vi "H5Literate_by_name.vi"(0 "Location Ref":T1, 1 "Index Type":T3 items=["H5_INDEX_UNKNOWN"=-1, "H5_INDEX_NAME"=0, "H5_INDEX_CRT_ORDER"=1], 2 "Order":T2 items=["H5_ITER_UNKNOWN"=-1, "H5_ITER_INC"=0, "H5_ITER_DEC"=1], 5 "Name":string=".", 7 "User data":variant, 9 "Index":u64, 11 "error in (no error)":errorcluster, 12 "Callback VI Ref":refnum<vi>, 13 "lapl_id":T1) -> (4 "Location Ref out":T1, 8 "User data out":variant, 10 "Index out":u64, 15 "error out":errorcluster)   [LabVIEW 2017]
doc: "Iterates through links in a group."
uses:
  <vilib>/UPVI/lvhdf5/library.llb/HDF5 Ref.ctl
  <vilib>/UPVI/lvhdf5/link.llb/H5L_info_t.ctl
  <vilib>/UPVI/lvhdf5/link.llb/H5L_type_t.ctl
  <vilib>/UPVI/lvhdf5/datatype.llb/H5T_cset_t.ctl
  <vilib>/UPVI/lvhdf5/library.llb/H5_index_t.ctl
  <vilib>/UPVI/lvhdf5/library.llb/H5_iter_order_t.ctl
  <vilib>/UPVI/lvhdf5/h5helper.dll
panel:
  in  "Event Data Type":T7 {"info"."cset" items=["H5T_CSET_ERROR"=-1, "H5T_CSET_ASCII"=0, "H5T_CSET_UTF8"=1]; "info"."type" items=["H5L_TYPE_ERROR"=-1, "H5L_TYPE_HARD"=0, "H5L_TYPE_SOFT"=1, "H5L_TYPE_EXTERNAL"=64, "H5L_TYPE_MAX"=255]}
  # "LVHDF5 Toolkit\nCopyright (c) 2005-2013 by Jason D. Sommerville\nCopyright (c) 2014-2015 by UPVI, LLC.\n\nThis use and distribution of this file is governed by the terms found in \nLICENSE.txt distributed with this toolkit and installed at\n <user.lib>\\_lvhdf5\\LICENSE.txt"
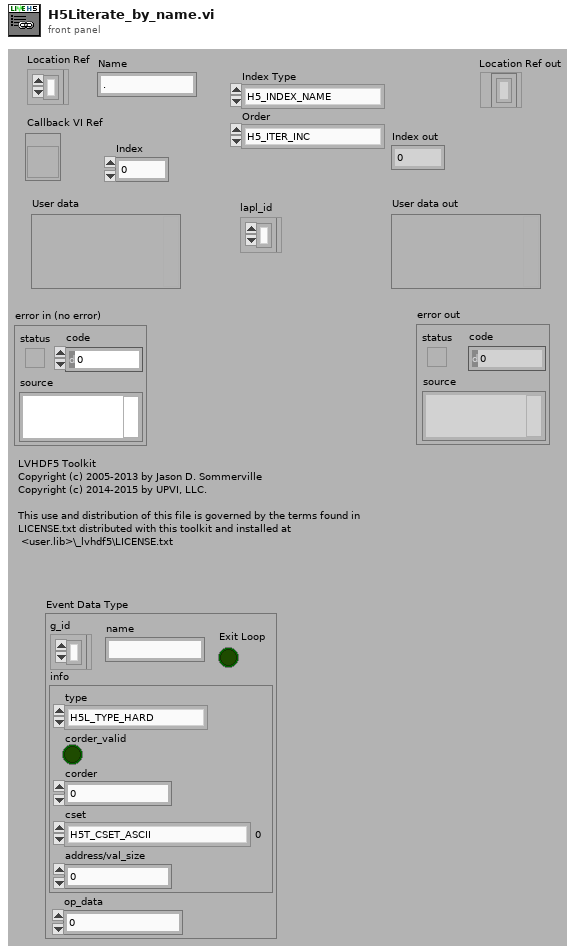
[diagram p1: front panel]
types:
  T1 = typedef "HDF5 Ref.ctl" = refnum<k1>
  T2 = typedef "H5_iter_order_t.ctl" = i32
  T3 = typedef "H5_index_t.ctl" = i32
  T4 = typedef "H5L_info_t.ctl" = cluster{"type":T5, "corder_valid":bool, "corder":i64, "cset":T6, "address/val_size":u64}
  T5 = typedef "H5L_type_t.ctl" = i32
  T6 = typedef "H5T_cset_t.ctl" = i32
  T7 = cluster{"g_id":T1, "name":string, "info":T4, "Exit Loop":bool, "op_data":u64}
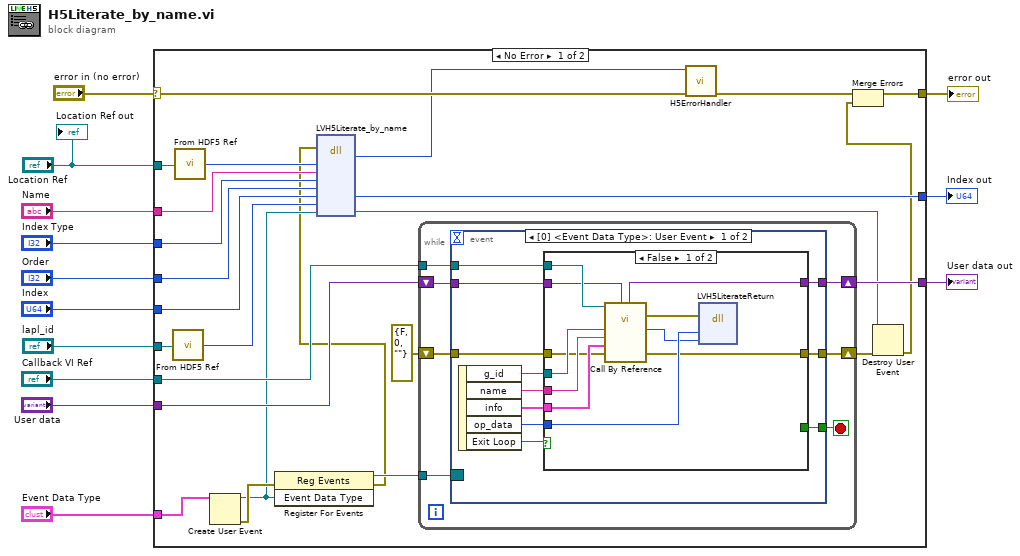
[diagram p0: block diagram]
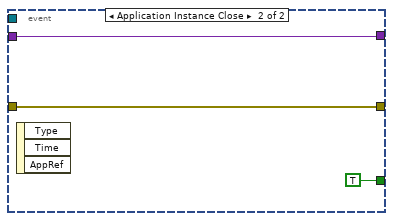
[diagram p3: hidden frame]
diagram:
  n1 = case shown="No Error" "error in (no error)" {
    selector: "error in (no error)" -> [w38 w76]
    tunnel: [w24 w76] -> w12
    tunnel: "Location Ref" -> [w36 _]
    tunnel: "Callback VI Ref" -> [w34 _]
    tunnel: "User data" -> [w33 w75]
    tunnel: "Event Data Type" -> [w30 _]
    tunnel: [w31 w75] -> w8
    tunnel: "Index" -> [w27 w74]
    tunnel: [w26 w74] -> w5
    tunnel: "Index Type" -> [w20 _]
    tunnel: "Order" -> [w19 _]
    tunnel: "Name" -> [w18 _]
    tunnel: "lapl_id" -> [w17 _]
    frame No Error {
      n2 = call <vilib>:"From HDF5 Ref.vi"("HDF5 Ref"=w17) -> ("I32"=w16:i32)
      n3 = call <vilib>:"From HDF5 Ref.vi"("HDF5 Ref"=w36) -> ("I32"=w28:i32)
      n4 = Create User Event(user event datatype=w30) -> (user event=w29:refnum<user-event>, error out=w35:errorcluster)  [unwired: 1 in]
      n5 = register-events(error in=w35, w29) -> (reference out=w32:refnum<event-registration>, error out=w15:errorcluster)  [unwired: 1 in]
      n6 = dll-call lib="C:/Program Files/National Instruments/LabVIEW 2017/vi.lib/UPVI/lvhdf5/h5helper.dll" fn="LVH5Literate_by_name"(error in=w15, "grp_id"=w28, "grp_name"=w18, "index_type"=w20, "order"=w19, "idx"=w27, "lapl_id"=w16, "lvevt"=w29) -> ("return type"=w37:i32, "idx"=w26:u64, "lvevt"=w21:refnum<user-event>)  [unwired: 7 in, 2 out]
      n7 = while {
        tunnel: w32 -> [w45]
        tunnel: w34 -> [w44]
        shift-right: [w42] -> w31
        shift-left: w33 -> [w43]
        shift-right: [w40] -> w23
        shift-left: errorcluster {"status"=FALSE, "code"=0, "source"=""} ("error out") -> [w39]
        stop <- w41 stop-if-true
        n8 = event shown="[0] <Event Data Type>: User Event" {
          selector: w45 -> [_ _]
          dyn-events: _ -> [_ _]
          timeout: _ -> [_ _]
          tunnel: w44 -> [w56 _]
          tunnel: w43 -> [w52 w72]
          tunnel: [w51 w72] -> w42
          tunnel: [w50 TRUE] -> w41
          tunnel: [w47 w71] -> w40
          tunnel: w39 -> [w46 w71]
          event User Event {
            n9 = event-data() -> ("g_id"=w55:T1, "name"=w54:string, "info"=w53:T4, "op_data"=w48:u64, "Exit Loop"=w49:bool)  [unwired: 1 in]
            n10 = case shown="False" w49 {
              selector: w49 -> [_ w69]
              tunnel: w56 -> [w67 _]
              tunnel: w55 -> [w66 _]
              tunnel: w54 -> [w65 _]
              tunnel: w53 -> [w64 _]
              tunnel: w52 -> [w63 w70]
              tunnel: [w62 w70] -> w51
              tunnel: [_ w69] -> w50
              tunnel: w48 -> [w60 _]
              tunnel: [w58 w68] -> w47
              tunnel: w46 -> [w57 w68]
              frame False {
                n11 = call-by-ref "?"(reference=w67, "op_data"=w63, "error in (no error)"=w57, "info"=w64, "name"=w65, "g_id"=w66) -> (error out=w61:errorcluster, 0:"error out"=w58:errorcluster, "Stop"=w59:i32, "op_data out"=w62:variant)  [unwired: 5 in, 1 out]
                n12 = dll-call lib="C:/Program Files/National Instruments/LabVIEW 2017/vi.lib/UPVI/lvhdf5/h5helper.dll" fn="LVH5LiterateReturn"(error in=w61, "op_data"=w60, "result"=w59) -> ()  [unwired: 5 in, 2 out]
              }
              frame True {
              }
            }
          }
          event Application Instance Close {
            n13 = event-data() -> ()  [unwired: 1 in, 3 out]
          }
        }
      }
      n14 = call <vilib>:"H5ErrorHandler.vi"("error in (no error)"=w38, "herr_t"=w37) -> ("error out"=w25:errorcluster)  [unwired: 3 in, 4 out]
      n15 = Destroy User Event(user event=w21, error in=w23) -> (error out=w22:errorcluster)
      n16 = Merge Errors(w25, w22) -> (w24:errorcluster)
    }
    frame Error {
    }
  }
  "error out" <- w12
  "User data out" <- w8
  "Index out" <- w5
  "Location Ref out" <- "Location Ref"
